vi "ep_Integration.vi"(3 "dt":dbl, 4 "state in":T2, 5 "x(t)":dbl[](array[numeric])) -> (1 "state out":T1, 2 "integrated x(t)":dbl[](array[numeric]))   [LabVIEW 2014, in "NI_EP_Motor Monitoring.lvlib"]
uses:
  <vilib>/addons/Electrical Power/Motor Monitoring/NI_EP_Motor Monitoring.lvlib
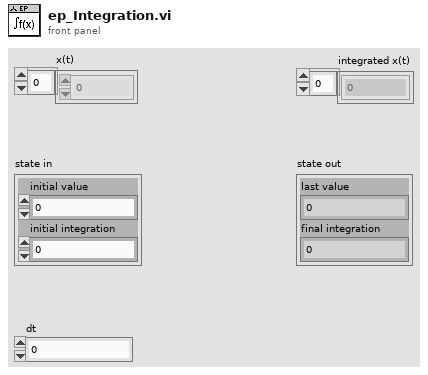
[diagram p1: front panel]
types:
  T1 = cluster{"last value":dbl, "final integration":dbl}
  T2 = cluster{"initial value":dbl, "initial integration":dbl}
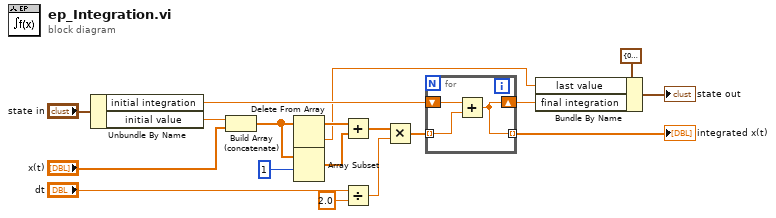
[diagram p0: block diagram]
diagram:
  n1 = Unbundle By Name("state in") -> ("initial integration"=w7:dbl, "initial value"=w17:dbl)
  n2 = Build Array (concatenate)(w17, "x(t)") -> (w15:dbl[])
  n3 = Delete From Array(array=w15) -> (deleted portion=w1:dbl, array with subset deleted=w13:dbl[])  [unwired: 2 in]
  n4 = Array Subset(array=w15, index=1) -> (w12:dbl[])  [unwired: 1 in]
  n5 = Add(x=w13, y=w12) -> (x+y=w11:dbl[])
  n6 = Divide(x="dt", y=2.0) -> (x/y=w8:dbl)
  n7 = Multiply(x=w11, y=w8) -> (x*y=w6:dbl[])
  n8 = for {
    shift-right: [w19] -> w3
    shift-left: w7 -> [w21]
    tunnel: w6 -> [w20] mode=indexing
    tunnel: [w19] -> w5 mode=indexing
    n9 = Add(x=w21, y=w20) -> (x+y=w19:dbl)
  }
  "integrated x(t)" <- w5
  n10 = Bundle By Name(cluster=T1 {"last value"=0.0, "final integration"=0.0} ("state out"), "last value"=w1, "final integration"=w3) -> (→"state out":T1)
